vi "Formula(Table).vi"(6 "式":T1, 8 "error in (no error)":errorcluster caption="エラー入力（エラーなし）", 9 "B値(列位置 0～)":u16, 10 "A値(列位置 0～)":u16, 11 "元データ(2D)":string[][](array[string])) -> (0 "error out":errorcluster caption="エラー出力", 3 "結果データ(1D)":dbl[](array[numeric]))   [LabVIEW 2014]
uses:
  EnumFormula.ctl
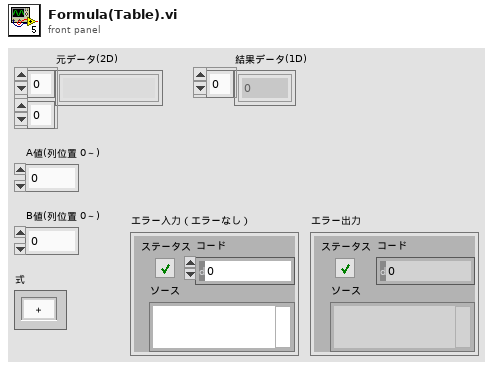
[diagram p1: front panel]
types:
  T1 = typedef "EnumFormula.ctl" = enum16{"＋", "－", "×"}
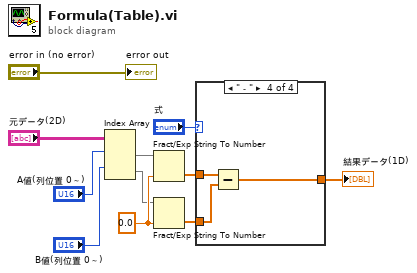
[diagram p0: block diagram]
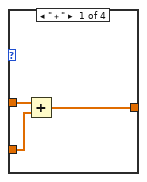
[diagram p2: hidden frame]
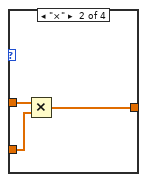
[diagram p3: hidden frame]
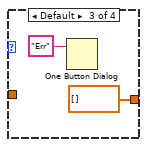
[diagram p4: hidden frame]
diagram:
  w7 = 0.0 ("デフォルト（0 I32）")
  n1 = Index Array(array="元データ(2D)", index (row) #1="A値(列位置 0～)", index (row) #2="B値(列位置 0～)") -> (element #1=w5:string[], element #2=w6:string[])  [unwired: 2 in]
  n2 = Fract/Exp String To Number(string=w5, default (0 dbl)=w7) -> (number=w9:dbl[])  [unwired: 2 in, 1 out]
  n3 = Fract/Exp String To Number(string=w6, default (0 dbl)=w7) -> (number=w8:dbl[])  [unwired: 2 in, 1 out]
  n4 = case shown="\"－\"" "式" {
    tunnel: w8 -> [w13 w16 _ w21]
    tunnel: w9 -> [w14 w17 _ w22]
    tunnel: [w12 w15 dbl[] [] w20] -> w10
    frame "＋" {
      # "足し算"
      n5 = Add(x=w14, y=w13) -> (x+y=w12:dbl[])
    }
    frame "×" {
      n6 = Multiply(x=w17, y=w16) -> (x*y=w15:dbl[])
    }
    frame Default {
      n7 = One Button Dialog(message="Err" ("メッセージ")) -> ()  [unwired: 1 in, 1 out]
    }
    frame "－" {
      # "引き算"
      n8 = Subtract(x=w22, y=w21) -> (x-y=w20:dbl[])
    }
  }
  "結果データ(1D)" <- w10
  "error out" <- "error in (no error)"
